vi "Set Reason.vi"(4 "Reasons":string[](array[string]), 6 "Codes":i32[](array[numeric]), 10 "error in (no error)":errorcluster) -> (2 "error out":errorcluster)   [LabVIEW 2020, in "Multiple Errors.lvclass"]
uses:
  Multiple Errors.lvclass
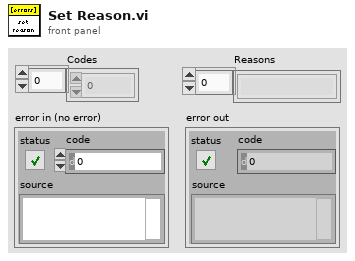
[diagram p1: front panel]
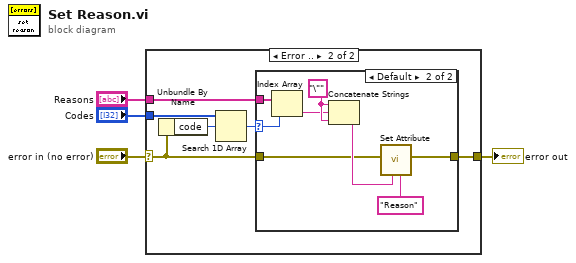
[diagram p0: block diagram]
diagram:
  n1 = case shown="Error .." "error in (no error)" {
    selector: "error in (no error)" -> [w5 w7]
    tunnel: [w5 w11] -> w3
    tunnel: "Reasons" -> [_ w6]
    tunnel: "Codes" -> [_ w9]
    frame No Error {
    }
    frame Error {
      n2 = Unbundle By Name(w7) -> ("code"=w10:i32)
      n3 = Search 1D Array(1D array=w9, element=w10) -> (index of element=w8:i32)  [unwired: 1 in]
      n4 = case shown="Default" w8 {
        selector: w8 -> [_ w14]
        tunnel: [w12 w20] -> w11
        tunnel: w7 -> [w12 w16]
        tunnel: w6 -> [_ w15]
        frame -1 {
        }
        frame Default {
          w18 = "\"" ("string")
          n5 = Index Array(array=w15, index=w14) -> (element=w13:string)
          n6 = Concatenate Strings(w18, w13, w18) -> (w19:string)
          n7 = call "Set Attribute.vi"("Attribute [\"Info\"]"="Reason" ("attribute name"), "Text"=w19, "error in (no error)"=w16) -> ("error out"=w20:errorcluster)  [unwired: 8 in]
        }
      }
    }
  }
  "error out" <- w3
